vi "addLockinClass.vi"(8 "error in (no error)":errorcluster, 10 "system.lvclass":refnum<class "system.lvclass">, 11 "UI_Main in":refnum<class "UI_Main.lvclass">) -> (0 "error out":errorcluster, 3 "UI_Main out":refnum<class "UI_Main.lvclass">)   [LabVIEW 2019, in "UI_Main.lvclass"]
uses:
  UI_Main.lvclass
  <vilib>/JKI/JKI SMO/SMO/SMO.lvclass
  lockin/system.lvclass
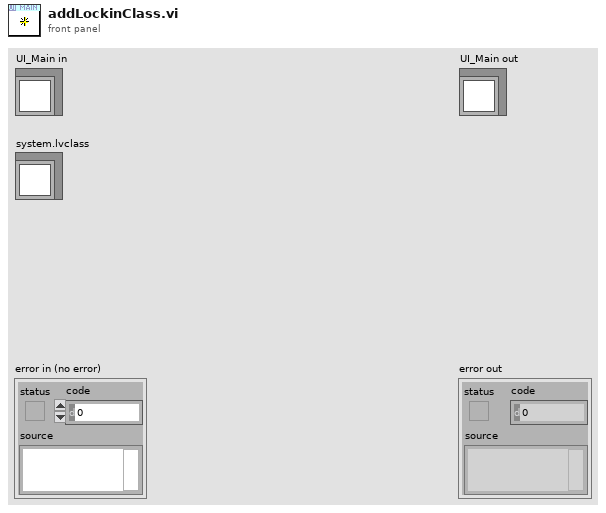
[diagram p1: front panel]
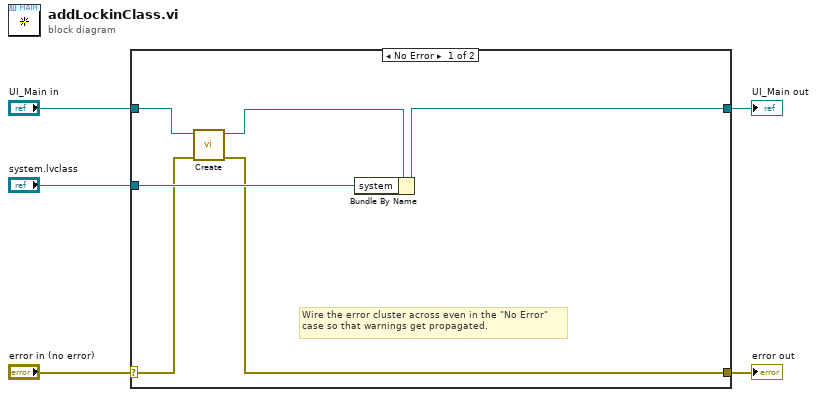
[diagram p0: block diagram]
diagram:
  n1 = case shown="No Error" "error in (no error)" {
    selector: "error in (no error)" -> [w7 w13]
    tunnel: [w6 w13] -> w4
    tunnel: [w11 w12] -> w2
    tunnel: "UI_Main in" -> [w9 w12]
    tunnel: "system.lvclass" -> [w10 _]
    frame No Error {
      # "Wire the error cluster across even in the \"No Error\"\ncase so that warnings get propagated."
      n2 = call <vilib>:"Create.vi"("error in (no error)"=w7, "SMO"=w9) -> ("error out"=w6:errorcluster, "SMO out"=w8:refnum<class "UI_Main.lvclass">)  [unwired: 7 in, 1 out]
      n3 = Bundle By Name(cluster=w8, "system"=w10) -> (w11:refnum<class "UI_Main.lvclass">)
    }
    frame Error {
    }
  }
  "error out" <- w4
  "UI_Main out" <- w2
